vi "Load Sub Panel.vi"(8 "error in (no error)":errorcluster, 10 "sub panel ref":refnum<vi>, 11 "View Cfg Base Template in":refnum<class "[V] Sys Cfg Base.lvclass">) -> (0 "error out":errorcluster, 3 "View Cfg Base Template out":refnum<class "[V] Sys Cfg Base.lvclass">)   [LabVIEW 2023, in "[V] Sys Cfg Base.lvlib" / "[V] Sys Cfg Base.lvclass"]
uses:
  [V] Sys Cfg Base.lvclass
  [V] Sys Cfg Base.lvclass/[V] Sys Cfg Base.ctl
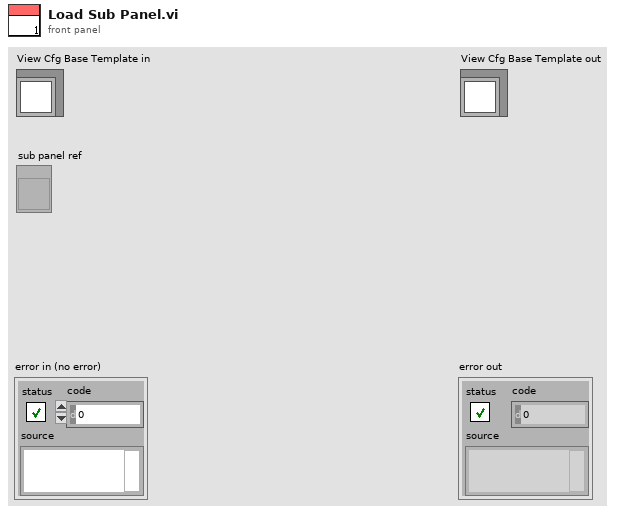
[diagram p1: front panel]
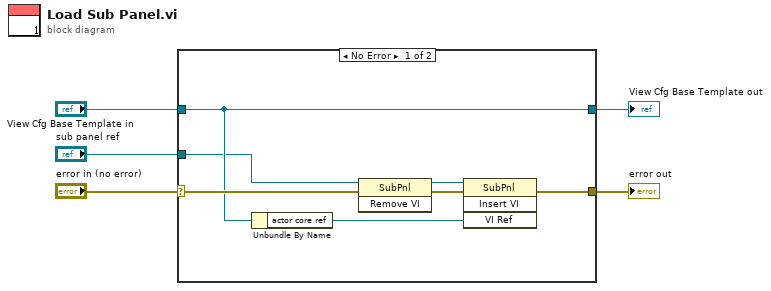
[diagram p0: block diagram]
diagram:
  n1 = case shown="No Error" "error in (no error)" {
    selector: "error in (no error)" -> [w9 w14]
    tunnel: [w10 w14] -> w4
    tunnel: [w7 w13] -> w2
    tunnel: "View Cfg Base Template in" -> [w7 w13]
    tunnel: "sub panel ref" -> [w6 _]
    frame No Error {
      n2 = Unbundle By Name(w7) -> ("actor core ref"=w8:refnum<vi>)
      n3 = invoke class="SubPnl" method="Remove VI"(reference=w6, error in=w9) -> (reference out=w11:refnum<vi>, error out=w12:errorcluster)  [unwired: 1 in, 1 out]
      n4 = invoke class="SubPnl" method="Insert VI"(reference=w11, error in=w12, "VI Ref"=w8) -> (error out=w10:errorcluster)  [unwired: 1 in, 3 out]
    }
    frame Error {
    }
  }
  "error out" <- w4
  "View Cfg Base Template out" <- w2
